vi "Trapezoidal Profile Lookup Setpoints.vi"(10 "Total Distance":sgl, 11 "Current Time":u32) -> (2 "Acceleration":sgl, 3 "Velocity":sgl, 4 "Profile Completed?":bool, 5 "Projected Current Distance":dbl)   [LabVIEW 2015]
uses:
  Trapezoidal Motion State.ctl
  Common Code/Change Detect Int.vi
  Robot Code/Robot Global Data.vi
panel:
  out "Stage 2 Time":sgl
  out "Stage 3 Time":sgl
  out "Stage 1 Time":sgl
  out "Max Reachable Velocity":sgl
  out "Cruise Velocity":sgl
  out "Total Time":sgl
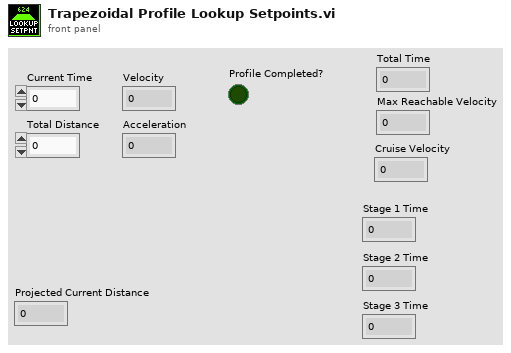
[diagram p1: front panel]
types:
  T1 = typedef "Trapezoidal Motion State.ctl" = enum16{"Accelerate", "Cruise", "Decelerate", "Finish"}
  T2 = typedef "Drivetrain Commands.ctl" = cluster{"Y Power":dbl, "Turn Power":dbl, "1st Gear?":bool, "Modes":T3, "Heading Target":dbl, "X Max Speed":dbl, "Y Max Speed":dbl, "X Min Speed":dbl, "Y Min Speed":dbl, "Y Target":dbl, "Max Accel":dbl, "Max Velocity":dbl}
  T3 = typedef "Drivetrain Modes.ctl" = enum16{"Climb", "Manual", "Vision Targeting", "PID Distance Drive", "Hybrid"}
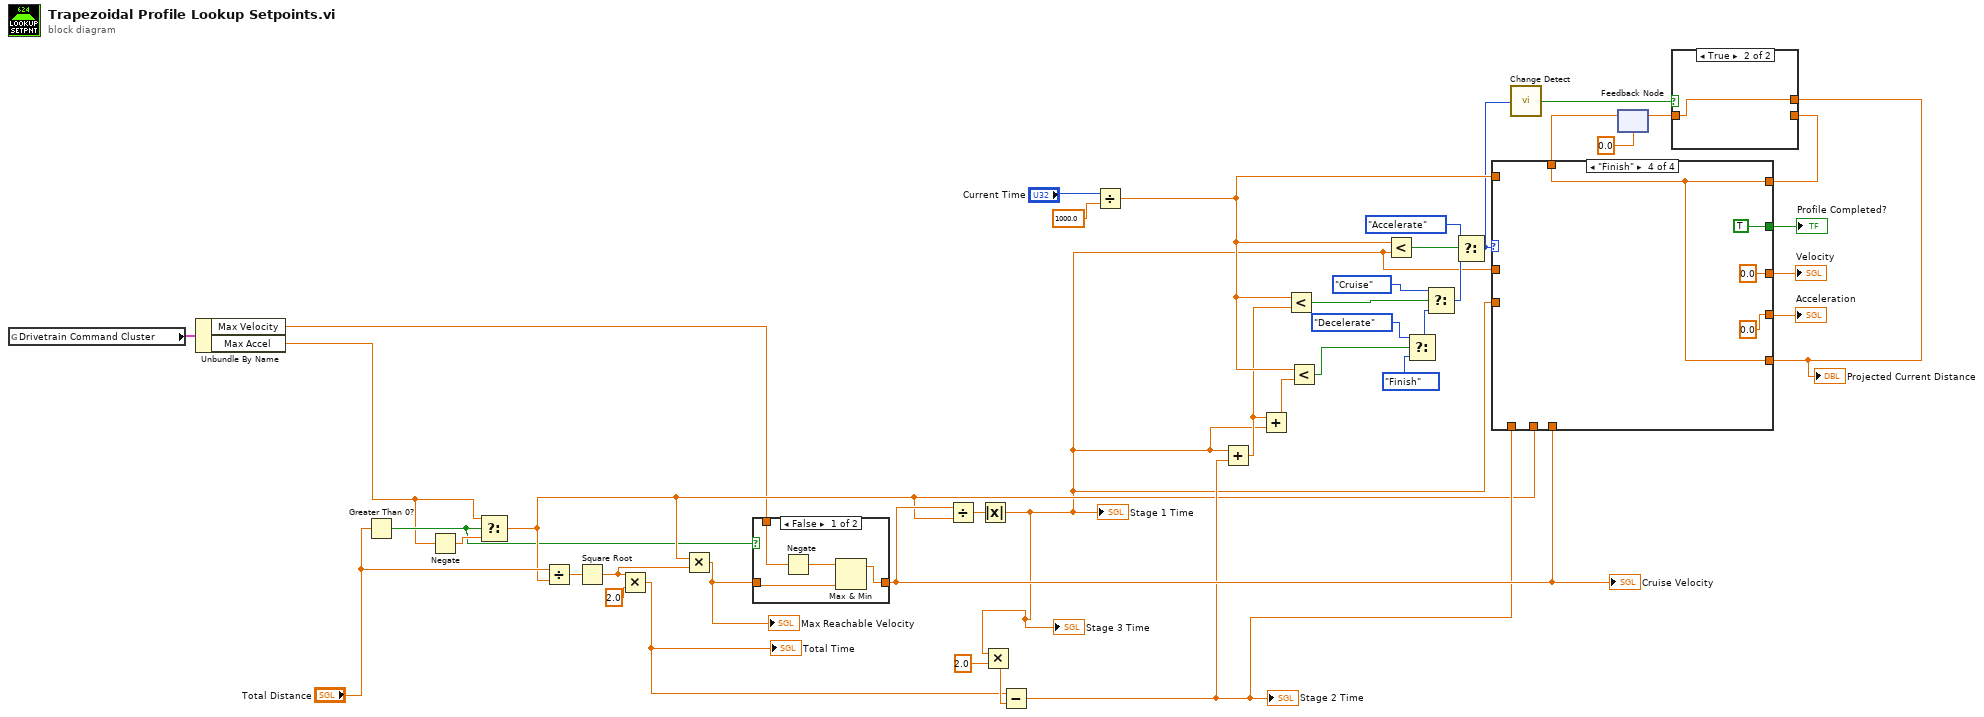
[diagram p0: block diagram]
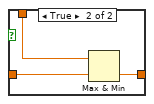
[diagram p3: hidden frame]
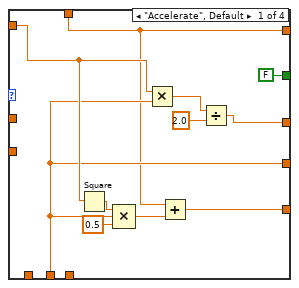
[diagram p4: hidden frame]
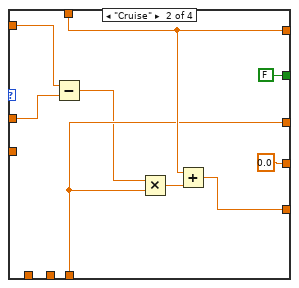
[diagram p5: hidden frame]
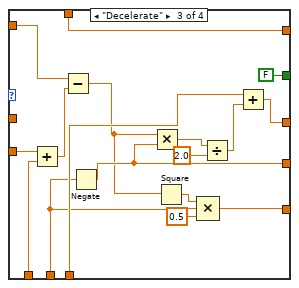
[diagram p6: hidden frame]
diagram:
  n1 = global read "Robot Global Data.vi" "Drivetrain Command Cluster"() -> (w3:T2)
  n2 = Unbundle By Name(w3) -> ("Max Velocity"=w1:dbl, "Max Accel"=w2:dbl)
  n3 = Greater Than 0?(x="Total Distance") -> (x > 0?=w13:bool)
  n4 = Negate(x=w2) -> (-x=w15:dbl)
  n5 = Select(t=w2, s=w13, f=w15) -> (s? t:f=w14:dbl)
  n6 = Divide(x="Total Distance", y=w14) -> (x/y=w31:dbl)
  n7 = Square Root(x=w31) -> (sqrt(x)=w29:dbl)
  n8 = Multiply(x=w29, y=sgl 2.0) -> (x*y=w22:dbl)
  "Total Time" <- w22
  n9 = Multiply(x=w14, y=w29) -> (x*y=w28:dbl)
  "Max Reachable Velocity" <- w28
  n10 = case shown="False" w13 {
    tunnel: w28 -> [w43 w49]
    tunnel: [w44 w48] -> w27
    tunnel: w1 -> [w46 w47]
    frame False {
      n11 = Negate(x=w46) -> (-x=w45:dbl)
      n12 = Max & Min(x=w45, y=w43) -> (max(x,y)=w44:dbl)  [unwired: 1 out]
    }
    frame True {
      n13 = Max & Min(x=w47, y=w49) -> (min(x,y)=w48:dbl)  [unwired: 1 out]
    }
  }
  "Cruise Velocity" <- w27
  n14 = Divide(x=w27, y=w14) -> (x/y=w12:dbl)
  n15 = Absolute Value(x=w12) -> (abs(x)=w4:dbl)
  "Stage 1 Time" <- w4
  "Stage 3 Time" <- w4
  n16 = Multiply(x=w4, y=sgl 2.0) -> (x*y=w25:dbl)
  n17 = Subtract(x=w22, y=w25) -> (x-y=w17:dbl)
  "Stage 2 Time" <- w17
  n18 = Divide(x="Current Time", y=sgl 1000.0) -> (x/y=w20:sgl)
  n19 = Add(x=w4, y=w17) -> (x+y=w19:dbl)
  n20 = Add(x=w19, y=w4) -> (x+y=w18:dbl)
  n21 = Less?(x=w20, y=w19) -> (x < y?=w40:bool)
  n22 = Less?(x=w20, y=w18) -> (x < y?=w37:bool)
  n23 = Less?(x=w20, y=w4) -> (x < y?=w42:bool)
  n24 = Select(t=Trapezoidal_Motion_State."Decelerate" ("Enum"), s=w37, f=Trapezoidal_Motion_State."Finish" ("Enum")) -> (s? t:f=w35:T1)
  n25 = Select(t=Trapezoidal_Motion_State."Cruise" ("Enum"), s=w40, f=w35) -> (s? t:f=w39:T1)
  n26 = Select(t=Trapezoidal_Motion_State."Accelerate" ("Enum"), s=w42, f=w39) -> (s? t:f=w11:T1)
  n27 = call-poly "Change Detect.vi"("In"=w11) -> ("Changed?"=w10:bool)
  n28 = feedback #1(sgl 0.0 ("Acceleration 3")) -> (w9:dbl)
  n29 = case shown="\"Finish\"" w11 {
    tunnel: [FALSE FALSE FALSE TRUE] -> w34
    tunnel: [w58 w65 w76 sgl 0.0 ("Cruise Velocity")] -> w33
    tunnel: [w54 sgl 0.0 ("Acceleration 3") w82 sgl 0.0 ("Acceleration 3")] -> w32
    tunnel: w20 -> [w55 w63 w86 _]
    tunnel: w27 -> [_ w65 w78 _]
    tunnel: w14 -> [w54 _ w72 _]
    tunnel: w17 -> [_ _ w80 _]
    tunnel: w4 -> [_ _ w81 _]
    tunnel: w9 -> [w50 w67 w75 w87]
    tunnel: [w50 w67 w75 w87] -> w6
    tunnel: [w51 w64 w70 w87] -> w5
    tunnel: w4 -> [_ w62 _ _]
    frame "Accelerate", Default {
      n30 = Square(x=w55) -> (x^2=w56:sgl)
      n31 = Compound Arithmetic op=MULTIPLY(w56, w54, 0.5 ("value")) -> (w52:dbl)
      n32 = Multiply(x=w55, y=w54) -> (x*y=w60:dbl)
      n33 = Add(x=w50, y=w52) -> (x+y=w51:dbl)
      n34 = Divide(x=w60, y=sgl 2.0) -> (x/y=w58:dbl)
    }
    frame "Cruise" {
      n35 = Subtract(x=w63, y=w62) -> (x-y=w61:dbl)
      n36 = Multiply(x=w61, y=w65) -> (x*y=w66:dbl)
      n37 = Add(x=w67, y=w66) -> (x+y=w64:dbl)
    }
    frame "Decelerate" {
      n38 = Add(x=w81, y=w80) -> (x+y=w79:dbl)
      n39 = Subtract(x=w86, y=w79) -> (x-y=w74:dbl)
      n40 = Negate(x=w72) -> (-x=w82:dbl)
      n41 = Multiply(x=w74, y=w82) -> (x*y=w85:dbl)
      n42 = Square(x=w74) -> (x^2=w73:dbl)
      n43 = Compound Arithmetic op=MULTIPLY(w73, w72, 0.5 ("value")) -> (w70:dbl)
      n44 = Divide(x=w85, y=sgl 2.0) -> (x/y=w77:dbl)
      n45 = Add(x=w78, y=w77) -> (x+y=w76:dbl)
    }
    frame "Finish" {
    }
  }
  "Velocity" <- w33
  "Acceleration" <- w32
  "Profile Completed?" <- w34
  "Projected Current Distance" <- w5
  n46 = case shown="True" w10 {
    tunnel: [w91 w92] -> w7
    tunnel: w6 -> [w91 _]
    tunnel: w5 -> [_ w92]
    frame False {
    }
    frame True {
    }
  }
  n47 = feedback-in #1(w7) -> ()
